vi "Loop_HW.vi"   [LabVIEW 2017, in "Joystick.lvlib"]
uses:
  Joystick.lvlib
  <vilib>/Rock Robotics/WPI/Joystick/WPI_JoystickDeviceEnum.ctl
  Globals/Global_STOP.vi
  Globals/Global_HW Data.vi
types:
  T1 = typedef "WPI_JoystickDeviceEnum.ctl" = enum16{"USB 0", "USB 1", "USB 2", "USB 3", "USB 4", "USB 5"}
  T2 = typedef "WPI_JoystickDevRef.ctl" = cluster{"Device":T1}
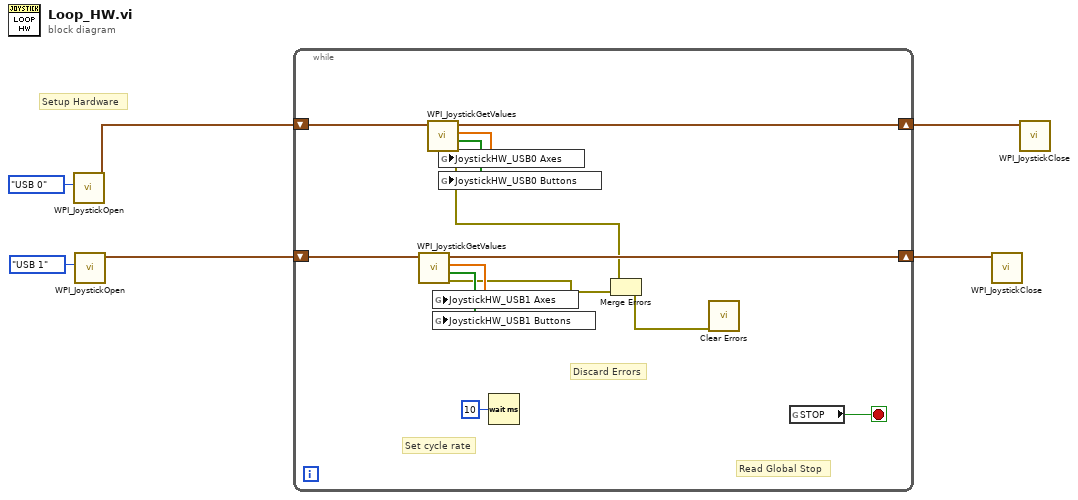
[diagram p0: block diagram]
diagram:
  # "Setup Hardware"
  n1 = call <vilib>:"WPI_JoystickOpen.vi"("JoystickDevice"=WPI_JoystickDeviceEnum."USB 0") -> ("JoystickDevRef"=w4:T2)  [unwired: 10 in]
  n2 = call <vilib>:"WPI_JoystickOpen.vi"("JoystickDevice"=WPI_JoystickDeviceEnum."USB 1") -> ("JoystickDevRef"=w3:T2)  [unwired: 10 in]
  n3 = while {
    shift-right: [w11] -> w2
    shift-left: w4 -> [w13]
    shift-right: [w10] -> w1
    shift-left: w3 -> [w12]
    stop <- w19 stop-if-true
    # "Discard Errors"
    # "Read Global Stop"
    # "Set cycle rate"
    n4 = call <vilib>:"WPI_JoystickGetValues.vi"("JoystickDevRef"=w12) -> ("error out"=w9:errorcluster, "Buttons"=w15:bool[], "Axes"=w14:dbl[], "JoystickDevRef"=w10:T2)  [unwired: 6 in, 1 out]
    n5 = call <vilib>:"WPI_JoystickGetValues.vi"("JoystickDevRef"=w13) -> ("error out"=w8:errorcluster, "Buttons"=w17:bool[], "Axes"=w16:dbl[], "JoystickDevRef"=w11:T2)  [unwired: 6 in, 1 out]
    n6 = global write "Global_HW Data.vi" "JoystickHW_USB1 Axes"(w14) -> ()
    n7 = global write "Global_HW Data.vi" "JoystickHW_USB1 Buttons"(w15) -> ()
    n8 = global write "Global_HW Data.vi" "JoystickHW_USB0 Axes"(w16) -> ()
    n9 = global write "Global_HW Data.vi" "JoystickHW_USB0 Buttons"(w17) -> ()
    n10 = Wait (ms)(milliseconds to wait=u32 10) -> ()  [unwired: 1 out]
    n11 = Merge Errors(w8, w9) -> (w7:errorcluster)
    n12 = call <vilib>:"Clear Errors.vi"("error in (no error)"=w7) -> ()  [unwired: 5 in, 2 out]
    n13 = global read "Global_STOP.vi" "STOP"() -> (w19:bool)
  }
  n14 = call <vilib>:"WPI_JoystickClose.vi"("JoystickDevRef"=w1) -> ()  [unwired: 11 in]
  n15 = call <vilib>:"WPI_JoystickClose.vi"("JoystickDevRef"=w2) -> ()  [unwired: 11 in]
